vi "导出曲线数组.vi"(0 "压轴承位移参数":dbl[](array[numeric]), 1 "压轴承压力参数":dbl[](array[numeric]), 2 "压衬套位移参数":dbl[](array[numeric]), 3 "压垫片位移参数":dbl[](array[numeric]), 4 "压垫片压力参数":dbl[](array[numeric]), 5 "压衬套力参数":dbl[](array[numeric]), 7 "file path (dialog if empty)":path caption="文件路径 （空时为对话框）") -> ()   [LabVIEW 2013]
uses:
  <vilib>/Utility/file.llb/Write To Spreadsheet File (DBL).vi
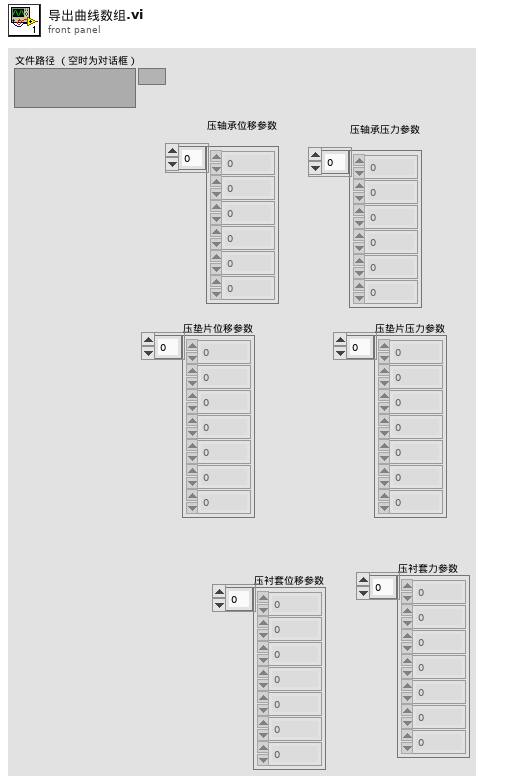
[diagram p1: front panel]
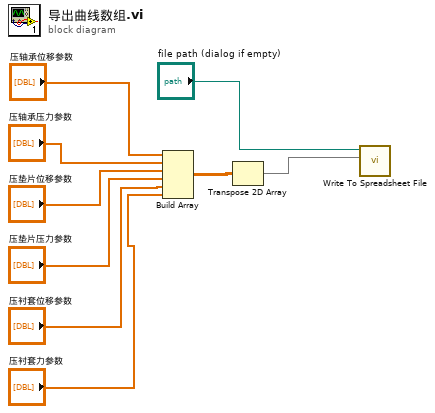
[diagram p0: block diagram]
diagram:
  n1 = Build Array("压轴承位移参数", "压轴承压力参数", "压垫片位移参数", "压垫片压力参数", "压衬套位移参数", "压衬套力参数") -> (w7:dbl[][])
  n2 = Transpose 2D Array(2D array=w7) -> (transposed array=w6:dbl[][])
  n3 = call-poly <vilib>:"Write To Spreadsheet File.vi"("2D data"=w6, "file path (dialog if empty)"="file path (dialog if empty)") -> ()  [unwired: 6 in, 1 out]
